vi "ellipse_lm_objective.vi"(3 "output control":T1, 4 "data":variant, 5 "X":dbl[](array[numeric]), 6 "a":dbl[](array[numeric])) -> (0 "error out":errorcluster, 1 "f'(X,a)":dbl[][](array[numeric]), 2 "f(X,a)":dbl[](array[numeric]))   [LabVIEW 2017]
doc: "This template is the starting point for creating a model function to be passed to the Nonlinear Curve Fit.vi."
uses:
  <vilib>/gmath/NumericalOptimization/LM_output select.ctl
  <vilib>/gmath/NI_Gmath.lvlib
panel:
  # "a[0] = a, a[1] = b, a[2] = theta, a[3] = B0"
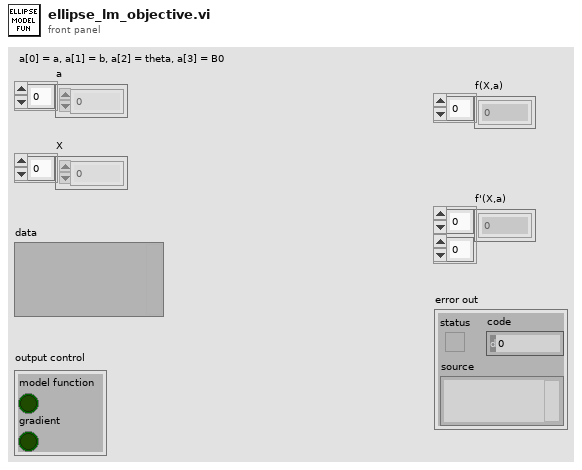
[diagram p1: front panel]
types:
  T1 = typedef "NI_Gmath.lvlib/LM_output select.ctl" = cluster{"model function":bool, "gradient":bool}
  T2 = cluster{"a[0]":dbl, "a[1]":dbl, "a[2]":dbl, "a[3]":dbl, "a[4]":dbl, "a[5]":dbl, "a[6]":dbl, "a[7]":dbl, "a[8]":dbl, "a[9]":dbl, "a[10]":dbl}
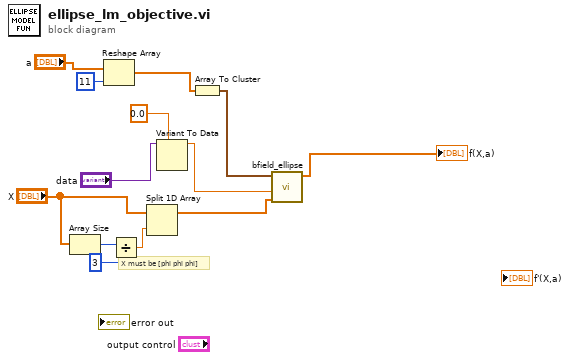
[diagram p0: block diagram]
diagram:
  # "X must be [phi phi phi]"
  n1 = Array Size(array="X") -> (size(s)=w12:i32)
  n2 = Reshape Array("a", 11 ("dimension size")) -> (w5:dbl[])
  n3 = Divide(x=w12, y=3) -> (x/y=w10:dbl)
  n4 = Split 1D Array(array="X", index=w10) -> (first subarray=w9:dbl[])  [unwired: 1 out]
  n5 = Variant To Data(type=0.0, Variant="data") -> (data=w2:dbl)  [unwired: 1 in, 1 out]
  n6 = Array To Cluster(array=w5) -> (cluster=w4:T2)
  n7 = call "bfield_ellipse.vi"("phi"=w9, "L"=w2, "parameters"=w4) -> ("B(a,phi) as 1D"=→"f(X,a)":dbl[])  [unwired: 8 in]
